vi "Legend Palette.vi"(4 "Active Plot":i32, 6 "Control Ref Queue":T1, 9 "Window Bounds":T5, 10 "Multiplot Representation In":T2, 11 "2D Error Bar.lvclass in":refnum<class "2D Error Bar.lvclass">) -> (1 "Cancel?":bool, 2 "Multiplot Representation Out":T2, 3 "2D Error Bar.lvclass out":refnum<class "2D Error Bar.lvclass">)   [LabVIEW 2020, in "2D Error Bar.lvclass"]
uses:
  <vilib>/Math Plots/2D Math Plots/2D Error Bar/2D Error Bar/2D Error Bar.lvclass
  <vilib>/Math Plots/2D Math Plots/2D Plot/2D Plot/Typedef/Multiplot Representation.ctl
  <vilib>/Math Plots/2D Math Plots/2D Plot/2D Plot/Typedef/Plot Representation.ctl
  <vilib>/Math Plots/2D Math Plots/2D Plot/2D Plot/Typedef/Range Cluster.ctl
  <vilib>/Math Plots/2D Math Plots/2D Plot/Action String/2DMathPlot Ctrl Act Queue.ctl
  <vilib>/Math Plots/2D Math Plots/2D Plot/Action String/2DMathPlot Ctrl Act Cluster.ctl
  <vilib>/Math Plots/2D Math Plots/2D Plot/Action String/2DMathPlot State Class.ctl
  e:/builds/penguin/labview/branches/2020/dev/dist/vi.lib/Math Plots/2D Math Plots/2D Plot/2D Plot/2D Plot.lvclass
  <vilib>/Utility/miscctls.llb/LVRectTypeDef.ctl
  <vilib>/Math Plots/2D Math Plots/2D Error Bar/2D Error Bar/2D Error Bar.lvclass/2D Error Bar.ctl
  <vilib>/Math Plots/2D Math Plots/2D Plot/2D Plot/2D Plot.lvclass
panel:
  in  "Tab Control":enum32{"Plot Property", "Input & Output"}(tab)
  in  "Fill To":u16(ring) caption="Line width"
  in  "Marker Style":u16(ring) caption="Line style"
  in  "Marker Width":u16(ring) caption="Line width"
  in  "Fill Color":u32(colorbox)
  in  "Fill Style":u16(ring) caption="Line style"
  in  "Point Style":u16(ring) caption="Line width"
  in  "Line Color":u32(colorbox)
  in  "Marker Color":u32(colorbox)
  in  "Marker Size":dbl caption="Error Bar size"
  in  "Cancel":bool
  in  "OK":bool
  in  "Line Style":u16(ring) caption="Line style"
  in  "Line Width":u16(ring) caption="Line width"
  # "Line style"
  # "Line width"
  # "Line color"
  # "Point style"
  # "Fill style"
  # "Fill to"
  # "Point/fill color"
  # "Marker width"
  # "Marker style"
  # "Marker color"
  # "Marker size"
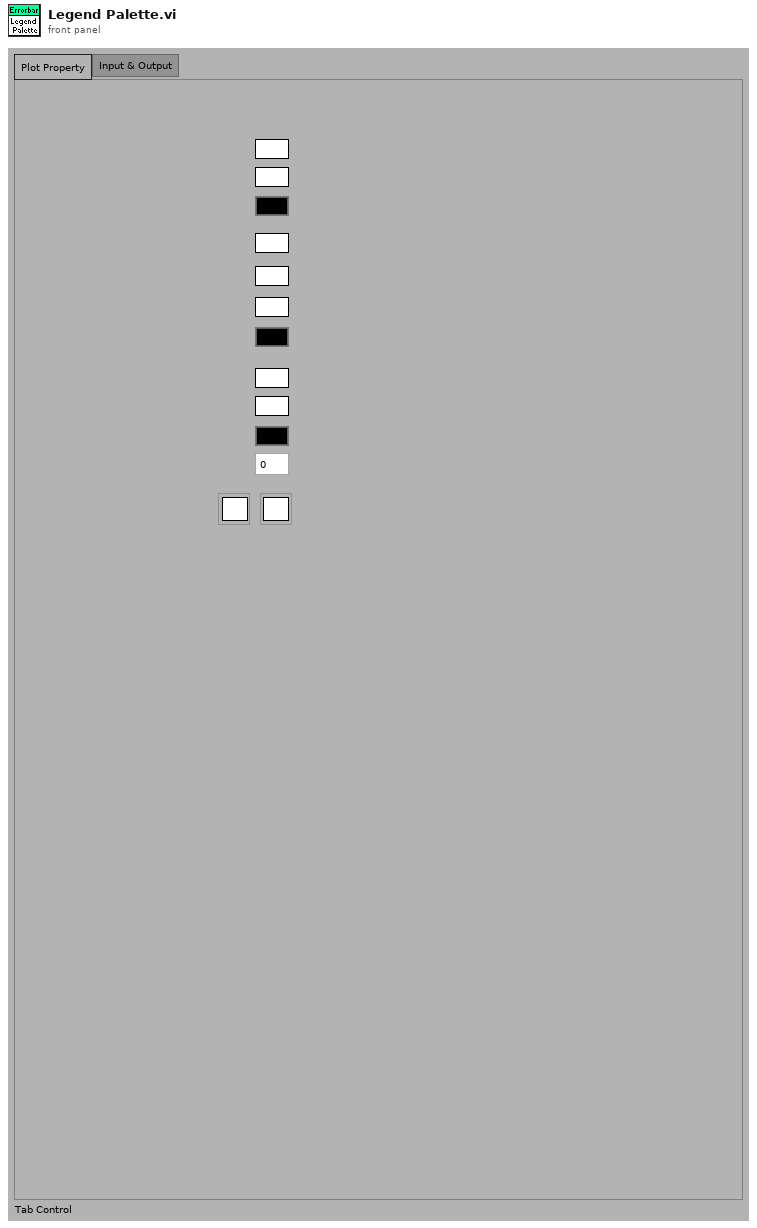
[diagram p1: front panel]
types:
  T1 = typedef "2DMathPlot Ctrl Act Queue.ctl" = refnum<queue>
  T2 = typedef "2D Plot.lvclass/Multiplot Representation.ctl" = cluster{"Plot Representation Array":T3[], "Max Range":T4}
  T3 = typedef "2D Plot.lvclass/Plot Representation.ctl" = cluster{"Plot Range":T4, "Vertex Cluster":cluster{"Vertex X Array":dbl[], "Vertex Y Array":dbl[]}, "Base Cluster":cluster{"Base X Array":dbl[], "Base Y Array":dbl[]}}
  T4 = typedef "2D Plot.lvclass/Range Cluster.ctl" = cluster{"X Range":cluster{"Max X":dbl, "Min X":dbl}, "Y Range":cluster{"Max Y":dbl, "Min Y":dbl}}
  T5 = typedef "LVRectTypeDef.ctl" = cluster{"Left":i16, "Top":i16, "Right":i16, "Bottom":i16}
  T6 = typedef "2DMathPlot Ctrl Act Cluster.ctl" = cluster{"Plot Area Ref":refnum<vi>, "Z Axis Ref":refnum<vi>, "Legend Ref":refnum<vi>, "XControl Ref":refnum<vi>, "Facade Ref":refnum<vi>, "Display State Change Class":T7}
  T7 = typedef "2DMathPlot State Class.ctl" = enum16{"Update All (Undo)", "Update General", "Update Appearance", "Update Format", "Update Scale", "Update Marker", "Update Cursor", "None"}
  T8 = typedef "2D Plot.lvclass/Plot Property Array.ctl" = T9[]
  T9 = typedef "2D Plot.lvclass/Plot Property.ctl" = cluster{"Bar Plot Style":u8, "DigitalLineStyle":u8, "TransitionLocation":u8, "Transition Type":u8, "Fill To":i16, "Fill/Pt. Color":u32, "Label Style":u8, "Line Style":u8, "Line Width":u8, "Plot Color":u32, "Plot Interpolation":u8, "Plot Name":string, "Point Style":u8, "Visible?":bool, "XScaleIdx":u32, "YScaleIdx":u32}
  T10 = typedef "2D Error Bar.lvclass/2D Error Bar Property Array.ctl" = T11[]
  T11 = typedef "2D Error Bar.lvclass/2D Error Bar Property.ctl" = cluster{"Marker Size":dbl, "Marker Line Style":u8, "Marker Line Width":u8, "Marker Color":u32, "Error Bar Interpolation":enum16{"Show Point", "Show Line", "Show Bar"}, "Error Mode":enum16{"Show Y Error", "Show X Error", "Show Both Error"}}
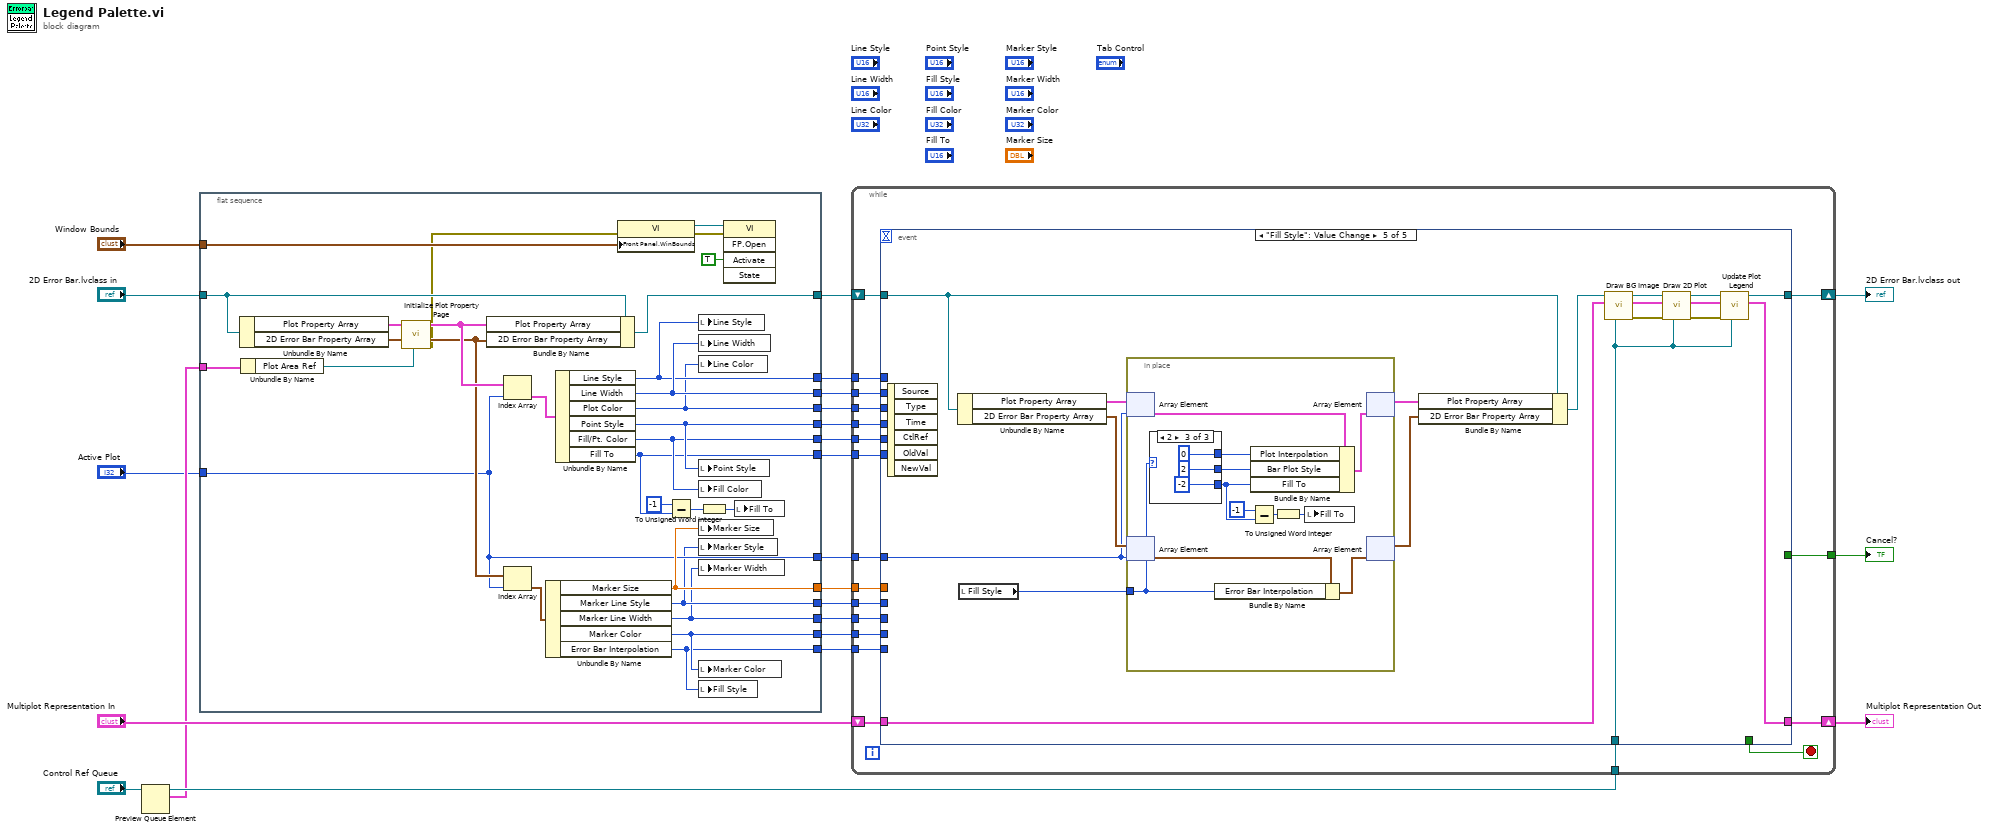
[diagram p0: block diagram]
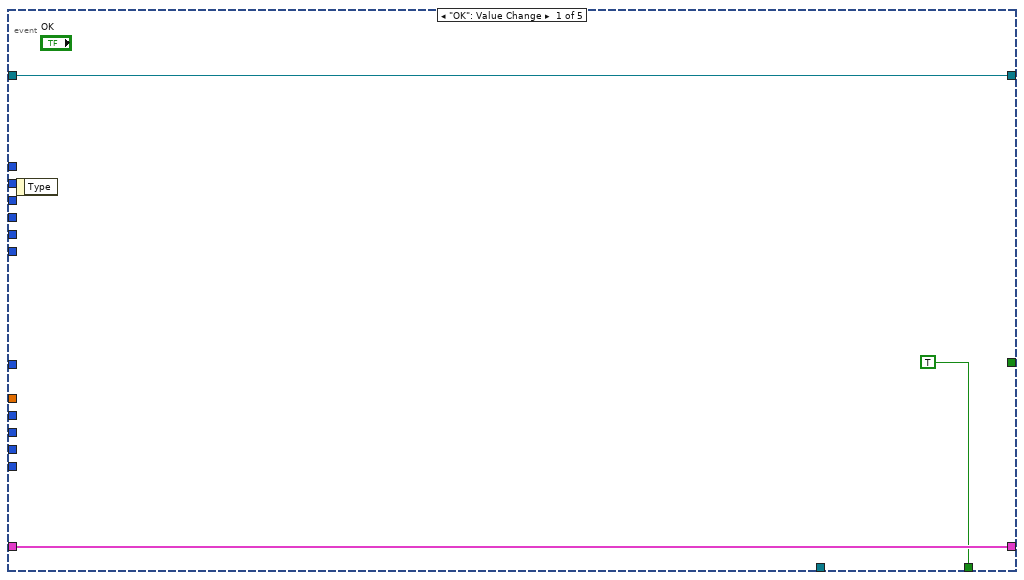
[diagram p2: hidden frame]
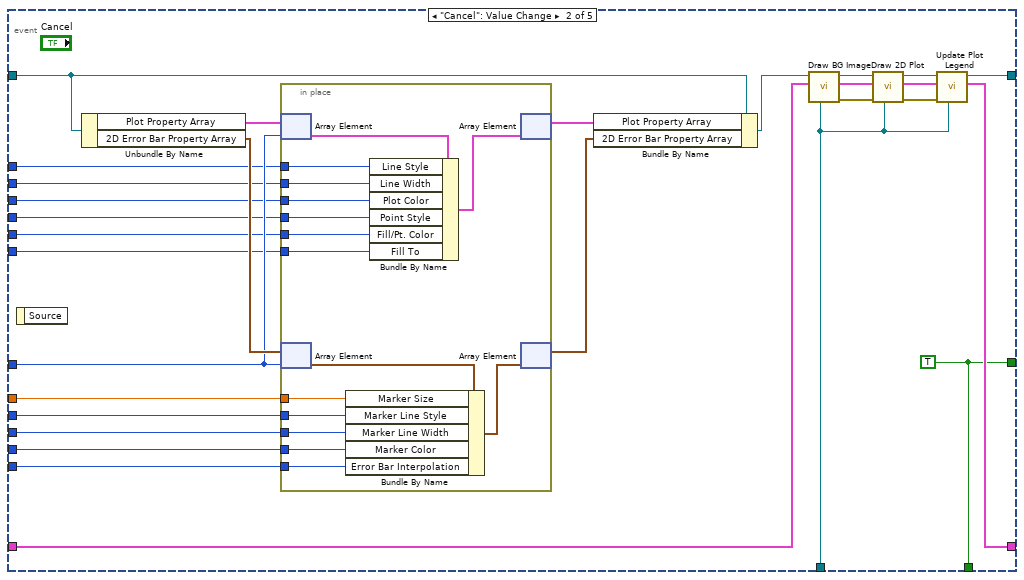
[diagram p3: hidden frame]
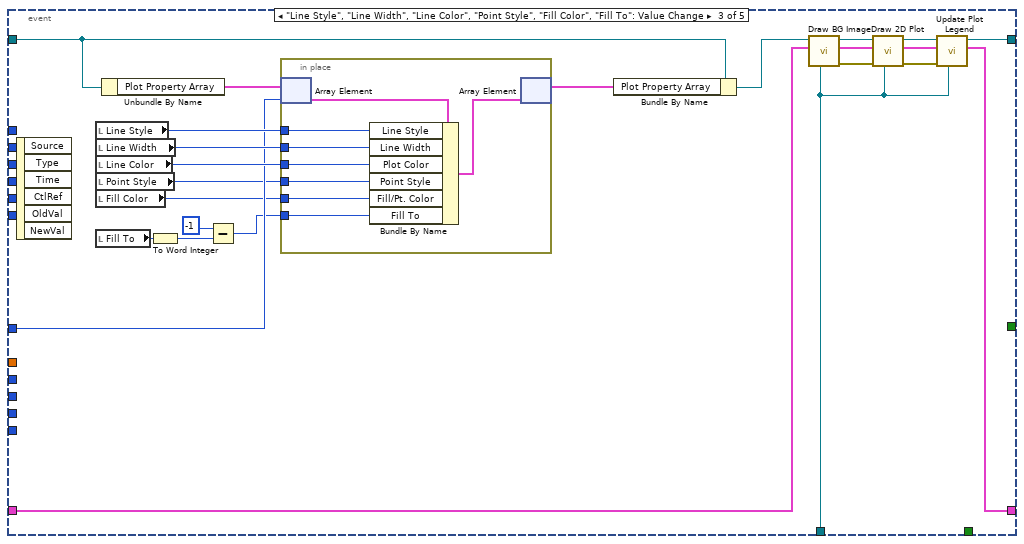
[diagram p4: hidden frame]
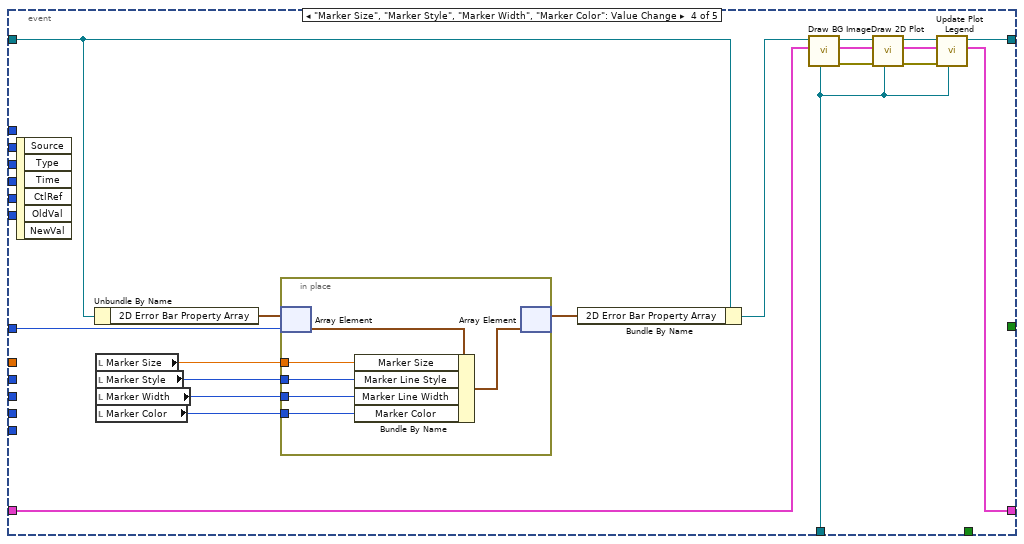
[diagram p5: hidden frame]
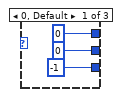
[diagram p6: hidden frame]
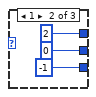
[diagram p7: hidden frame]
diagram:
  n1 = Preview Queue Element(queue="Control Ref Queue") -> (queue out=w17:T1, element=w16:T6)  [unwired: 1 in, 3 out]
  n2 = flat-sequence {
    tunnel: "2D Error Bar.lvclass in" -> [w43]
    tunnel: [w42] -> w21
    tunnel: [w38] -> w11
    tunnel: w16 -> [w51]
    tunnel: [w50] -> w15
    tunnel: [w37] -> w14
    tunnel: [w49] -> w13
    tunnel: [w48] -> w12
    tunnel: "Window Bounds" -> [w40]
    tunnel: "Active Plot" -> [w38]
    tunnel: [w36] -> w7
    tunnel: [w35] -> w6
    tunnel: [w29] -> w5
    tunnel: [w34] -> w4
    tunnel: [w33] -> w3
    tunnel: [w32] -> w2
    tunnel: [w31] -> w1
    frame #0 {
      n3 = Unbundle By Name(w43) -> ("Plot Property Array"=w47:T8, "2D Error Bar Property Array"=w46:T10)
      n4 = Unbundle By Name(w51) -> ("Plot Area Ref"=w41:refnum<vi>)
      n5 = call <vilib>:"Initialize Plot Property Page.vi"("Plot Area Ref"=w41, "2D Error Bar Array In"=w46, "Plot Property Array In"=w47) -> ("error out"=w39:errorcluster, "2D Error Bar Array Out"=w44:T10, "Plot Property Array Out"=w45:T8)  [unwired: 2 in, 4 out]
      n6 = Bundle By Name(cluster=w43, "Plot Property Array"=w45, "2D Error Bar Property Array"=w44) -> (w42:refnum<class "2D Error Bar.lvclass">)
      n7 = Index Array(array=w45, index=w38) -> (element=w53:T9)
      n8 = Index Array(array=w44, index=w38) -> (element=w52:T11)
      n9 = Unbundle By Name(w52) -> ("Marker Size"=w50:dbl, "Marker Line Style"=w34:u8, "Marker Line Width"=w33:u8, "Marker Color"=w32:u32, "Error Bar Interpolation"=w31:enum16{"Show Point", "Show Line", "Show Bar"})
      n10 = Unbundle By Name(w53) -> ("Line Style"=w48:u8, "Line Width"=w49:u8, "Plot Color"=w37:u32, "Point Style"=w36:u8, "Fill/Pt. Color"=w35:u32, "Fill To"=w29:i16)
      n11 = property class="VI"(error in=w39, "Front Panel.WinBounds"=w40) -> (reference out=w26:refnum<vi>, error out=w25:errorcluster)  [unwired: 1 in]
      n12 = Subtract(x=i16 -1, y=w29) -> (x-y=w28:i16)
      n13 = local write "Line Style"(w48) -> ()
      n14 = local write "Line Width"(w49) -> ()
      n15 = local write "Line Color"(w37) -> ()
      n16 = local write "Point Style"(w36) -> ()
      n17 = local write "Fill Color"(w35) -> ()
      n18 = local write "Marker Size"(w50) -> ()
      n19 = local write "Marker Style"(w34) -> ()
      n20 = local write "Marker Width"(w33) -> ()
      n21 = local write "Marker Color"(w32) -> ()
      n22 = local write "Fill Style"(w31) -> ()
      n23 = To Unsigned Word Integer(number=w28) -> (unsigned 16bit integer=w27:u16)
      n24 = invoke class="VI" method="FP.Open"(reference=w26, error in=w25, "Activate"=TRUE ("Activate?")) -> ()  [unwired: 2 in, 5 out]
      n25 = local write "Fill To"(w27) -> ()
    }
  }
  n26 = while {
    shift-right: [w71] -> w23
    shift-left: w21 -> [w72]
    shift-right: [w69] -> w19
    shift-left: "Multiplot Representation In" -> [w70]
    tunnel: w17 -> [w68]
    tunnel: w11 -> [w67]
    tunnel: w15 -> [w65]
    tunnel: w14 -> [w64]
    tunnel: w13 -> [w63]
    tunnel: w12 -> [w62]
    tunnel: [w61] -> w10
    tunnel: w7 -> [w60]
    tunnel: w6 -> [w59]
    tunnel: w5 -> [w58]
    tunnel: w4 -> [w57]
    tunnel: w3 -> [w56]
    tunnel: w2 -> [w55]
    tunnel: w1 -> [w54]
    stop <- w66 stop-if-true
    n27 = event shown="[4] \"Fill Style\": Value Change" {
      selector: _ -> [_ _ _ _ _]
      dyn-events: _ -> [_ _ _ _ _]
      timeout: _ -> [_ _ _ _ _]
      tunnel: w72 -> [w75 w99 w142 w169 w193]
      tunnel: [w75 w92 w134 w164 w189] -> w71
      tunnel: w70 -> [w74 w98 w136 w165 w190]
      tunnel: [w74 w91 w133 w163 w188] -> w69
      tunnel: w68 -> [_ w84 w126 w156 w181]
      tunnel: w67 -> [_ w97 w135 w152 w178]
      tunnel: [TRUE w83 _ _ _] -> w66
      tunnel: w65 -> [_ w96 _ _ _]
      tunnel: w64 -> [_ w95 _ _ _]
      tunnel: w63 -> [_ w94 _ _ _]
      tunnel: w62 -> [_ w93 _ _ _]
      tunnel: [_ w83 _ _ _] -> w61
      tunnel: w60 -> [_ w78 _ _ _]
      tunnel: w59 -> [_ w77 _ _ _]
      tunnel: w58 -> [_ w76 _ _ _]
      tunnel: w57 -> [_ w82 _ _ _]
      tunnel: w56 -> [_ w81 _ _ _]
      tunnel: w55 -> [_ w80 _ _ _]
      tunnel: w54 -> [_ w79 _ _ _]
      event "OK": Value Change {
        n28 = event-data() -> ()  [unwired: 2 out]
      }
      event "Cancel": Value Change {
        w83 = TRUE
        n29 = event-data() -> ()  [unwired: 2 out]
        n30 = Unbundle By Name(w99) -> ("Plot Property Array"=w104:T8, "2D Error Bar Property Array"=w103:T10)
        n31 = in-place {
          in-place-border: w96 -> [w115]
          in-place-border: w93 -> [w114]
          in-place-border: w94 -> [w113]
          in-place-border: w95 -> [w112]
          in-place-border: w82 -> [w111]
          in-place-border: w81 -> [w110]
          in-place-border: w80 -> [w109]
          in-place-border: w79 -> [w108]
          in-place-border: w78 -> [w107]
          in-place-border: w77 -> [w106]
          in-place-border: w76 -> [w105]
          n32 = in-place-array #1(w104, w97) -> (w119:T9)
          n33 = in-place-array #2(w103, w97) -> (w118:T11)
          n34 = Bundle By Name(cluster=w118, "Marker Size"=w115, "Marker Line Style"=w111, "Marker Line Width"=w110, "Marker Color"=w109, "Error Bar Interpolation"=w108) -> (w117:T11)
          n35 = Bundle By Name(cluster=w119, "Line Style"=w114, "Line Width"=w113, "Plot Color"=w112, "Point Style"=w107, "Fill/Pt. Color"=w106, "Fill To"=w105) -> (w116:T9)
          n36 = in-place-array #1(w116) -> (w102:T8)  [unwired: 1 out]
          n37 = in-place-array #2(w117) -> (w101:T10)  [unwired: 1 out]
        }
        n38 = Bundle By Name(cluster=w99, "Plot Property Array"=w102, "2D Error Bar Property Array"=w101) -> (w100:refnum<class "2D Error Bar.lvclass">)
        n39 = call-dynamic "Draw BG Image.vi"("Control Ref Queue"=w84, "Multiplot Representation In"=w98, "2D Error Bar.lvclass in"=w100) -> ("error out"=w90:errorcluster, "Multiplot Representation Out"=w89:T2, "2D Error Bar.lvclass out"=w88:refnum<class "2D Error Bar.lvclass">)  [unwired: 1 in, 5 out]
        n40 = call-dynamic "Draw 2D Plot.vi"("Control Ref Queue"=w84, "error in (no error)"=w90, "Multiplot Representation In"=w89, "2D Error Bar.lvclass in"=w88) -> ("error out"=w85:errorcluster, "Multiplot Representation Out"=w86:T2, "2D Error Bar.lvclass out"=w87:refnum<class "2D Error Bar.lvclass">)  [unwired: 5 out]
        n41 = call <vilib>:"Update Plot Legend.vi"("Control Ref Queue"=w84, "error in (no error)"=w85, "Multiplot Representation In"=w86, "2D Plot in"=w87) -> ("Multiplot Representation Out"=w91:T2, "2D Plot out"=w92:refnum<class "2D Error Bar.lvclass">)  [unwired: 6 out]
      }
      event "Line Style", "Line Width", "Line Color", "Point Style", "Fill Color", "Fill To": Value Change {
        n42 = event-data() -> ()  [unwired: 7 out]
        n43 = local read "Line Style"() -> (w140:u16)
        n44 = local read "Line Width"() -> (w139:u16)
        n45 = local read "Line Color"() -> (w138:u32)
        n46 = local read "Point Style"() -> (w125:u16)
        n47 = local read "Fill Color"() -> (w124:u32)
        n48 = local read "Fill To"() -> (w122:u16)
        n49 = Unbundle By Name(w142) -> ("Plot Property Array"=w143:T8)
        n50 = To Word Integer(number=w122) -> (16bit integer=w120:i16)
        n51 = Subtract(x=i16 -1, y=w120) -> (x-y=w123:i16)
        n52 = in-place {
          in-place-border: w140 -> [w149]
          in-place-border: w139 -> [w148]
          in-place-border: w138 -> [w147]
          in-place-border: w125 -> [w146]
          in-place-border: w124 -> [w145]
          in-place-border: w123 -> [w144]
          n53 = in-place-array #3(w143, w135) -> (w151:T9)
          n54 = Bundle By Name(cluster=w151, "Line Style"=w149, "Line Width"=w148, "Plot Color"=w147, "Point Style"=w146, "Fill/Pt. Color"=w145, "Fill To"=w144) -> (w150:T9)
          n55 = in-place-array #3(w150) -> (w141:T8)  [unwired: 1 out]
        }
        n56 = Bundle By Name(cluster=w142, "Plot Property Array"=w141) -> (w137:refnum<class "2D Error Bar.lvclass">)
        n57 = call-dynamic "Draw BG Image.vi"("Control Ref Queue"=w126, "Multiplot Representation In"=w136, "2D Error Bar.lvclass in"=w137) -> ("error out"=w132:errorcluster, "Multiplot Representation Out"=w131:T2, "2D Error Bar.lvclass out"=w130:refnum<class "2D Error Bar.lvclass">)  [unwired: 1 in, 5 out]
        n58 = call-dynamic "Draw 2D Plot.vi"("Control Ref Queue"=w126, "error in (no error)"=w132, "Multiplot Representation In"=w131, "2D Error Bar.lvclass in"=w130) -> ("error out"=w127:errorcluster, "Multiplot Representation Out"=w128:T2, "2D Error Bar.lvclass out"=w129:refnum<class "2D Error Bar.lvclass">)  [unwired: 5 out]
        n59 = call <vilib>:"Update Plot Legend.vi"("Control Ref Queue"=w126, "error in (no error)"=w127, "Multiplot Representation In"=w128, "2D Plot in"=w129) -> ("Multiplot Representation Out"=w133:T2, "2D Plot out"=w134:refnum<class "2D Error Bar.lvclass">)  [unwired: 6 out]
      }
      event "Marker Size", "Marker Style", "Marker Width", "Marker Color": Value Change {
        n60 = event-data() -> ()  [unwired: 7 out]
        n61 = Unbundle By Name(w169) -> ("2D Error Bar Property Array"=w170:T10)
        n62 = local read "Marker Size"() -> (w167:dbl)
        n63 = local read "Marker Style"() -> (w155:u16)
        n64 = local read "Marker Width"() -> (w154:u16)
        n65 = local read "Marker Color"() -> (w153:u32)
        n66 = in-place {
          in-place-border: w167 -> [w174]
          in-place-border: w155 -> [w173]
          in-place-border: w154 -> [w172]
          in-place-border: w153 -> [w171]
          n67 = in-place-array #4(w170, w152) -> (w176:T11)
          n68 = Bundle By Name(cluster=w176, "Marker Size"=w174, "Marker Line Style"=w173, "Marker Line Width"=w172, "Marker Color"=w171) -> (w175:T11)
          n69 = in-place-array #4(w175) -> (w168:T10)  [unwired: 1 out]
        }
        n70 = Bundle By Name(cluster=w169, "2D Error Bar Property Array"=w168) -> (w166:refnum<class "2D Error Bar.lvclass">)
        n71 = call-dynamic "Draw BG Image.vi"("Control Ref Queue"=w156, "Multiplot Representation In"=w165, "2D Error Bar.lvclass in"=w166) -> ("error out"=w162:errorcluster, "Multiplot Representation Out"=w161:T2, "2D Error Bar.lvclass out"=w160:refnum<class "2D Error Bar.lvclass">)  [unwired: 1 in, 5 out]
        n72 = call-dynamic "Draw 2D Plot.vi"("Control Ref Queue"=w156, "error in (no error)"=w162, "Multiplot Representation In"=w161, "2D Error Bar.lvclass in"=w160) -> ("error out"=w157:errorcluster, "Multiplot Representation Out"=w158:T2, "2D Error Bar.lvclass out"=w159:refnum<class "2D Error Bar.lvclass">)  [unwired: 5 out]
        n73 = call <vilib>:"Update Plot Legend.vi"("Control Ref Queue"=w156, "error in (no error)"=w157, "Multiplot Representation In"=w158, "2D Plot in"=w159) -> ("Multiplot Representation Out"=w163:T2, "2D Plot out"=w164:refnum<class "2D Error Bar.lvclass">)  [unwired: 6 out]
      }
      event "Fill Style": Value Change {
        n74 = event-data() -> ()  [unwired: 7 out]
        n75 = Unbundle By Name(w193) -> ("Plot Property Array"=w180:T8, "2D Error Bar Property Array"=w194:T10)
        n76 = local read "Fill Style"() -> (w177:u16)
        n77 = in-place {
          in-place-border: w177 -> [w201]
          n78 = in-place-array #5(w180, w178) -> (w203:T9)
          n79 = in-place-array #6(w194, w178) -> (w205:T11)
          n80 = case shown="2" w201 {
            tunnel: [u8 0 ("Plot Interpolation") u8 2 ("Plot Interpolation") u8 0 ("Plot Interpolation")] -> w199
            tunnel: [u8 0 ("Plot Interpolation") u8 0 ("Plot Interpolation") u8 2 ("Plot Interpolation")] -> w200
            tunnel: [i16 -1 ("Fill To") i16 -1 ("Fill To") i16 -2 ("Fill To")] -> w196
            frame 0, Default {
            }
            frame 1 {
            }
            frame 2 {
            }
          }
          n81 = Bundle By Name(cluster=w205, "Error Bar Interpolation"=w201) -> (w204:T11)
          n82 = Bundle By Name(cluster=w203, "Plot Interpolation"=w199, "Bar Plot Style"=w200, "Fill To"=w196) -> (w202:T9)
          n83 = Subtract(x=i16 -1, y=w196) -> (x-y=w198:i16)
          n84 = To Unsigned Word Integer(number=w198) -> (unsigned 16bit integer=w195:u16)
          n85 = local write "Fill To"(w195) -> ()
          n86 = in-place-array #5(w202) -> (w179:T8)  [unwired: 1 out]
          n87 = in-place-array #6(w204) -> (w192:T10)  [unwired: 1 out]
        }
        n88 = Bundle By Name(cluster=w193, "Plot Property Array"=w179, "2D Error Bar Property Array"=w192) -> (w191:refnum<class "2D Error Bar.lvclass">)
        n89 = call-dynamic "Draw BG Image.vi"("Control Ref Queue"=w181, "Multiplot Representation In"=w190, "2D Error Bar.lvclass in"=w191) -> ("error out"=w187:errorcluster, "Multiplot Representation Out"=w186:T2, "2D Error Bar.lvclass out"=w185:refnum<class "2D Error Bar.lvclass">)  [unwired: 1 in, 5 out]
        n90 = call-dynamic "Draw 2D Plot.vi"("Control Ref Queue"=w181, "error in (no error)"=w187, "Multiplot Representation In"=w186, "2D Error Bar.lvclass in"=w185) -> ("error out"=w182:errorcluster, "Multiplot Representation Out"=w183:T2, "2D Error Bar.lvclass out"=w184:refnum<class "2D Error Bar.lvclass">)  [unwired: 5 out]
        n91 = call <vilib>:"Update Plot Legend.vi"("Control Ref Queue"=w181, "error in (no error)"=w182, "Multiplot Representation In"=w183, "2D Plot in"=w184) -> ("Multiplot Representation Out"=w188:T2, "2D Plot out"=w189:refnum<class "2D Error Bar.lvclass">)  [unwired: 6 out]
      }
    }
  }
  "2D Error Bar.lvclass out" <- w23
  "Multiplot Representation Out" <- w19
  "Cancel?" <- w10
